vi "DWF Dig Tristate Lines.vi"(0 "Instrument Handle In":u32, 5 "Lines":string, 11 "Error In":errorcluster caption="Error In (no error)") -> (4 "Instrument Handle Out":u32, 15 "Error Out":errorcluster)   [LabVIEW 2015, in "DigilentWF.lvlib"]
doc: "Sets all specified lines to a high-impedance state."
uses:
  <vilib>/DigilentWF/DigilentWF.lvlib
  dwf.dll
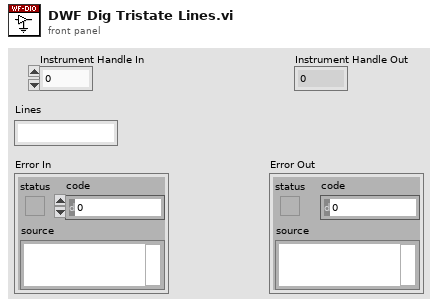
[diagram p1: front panel]
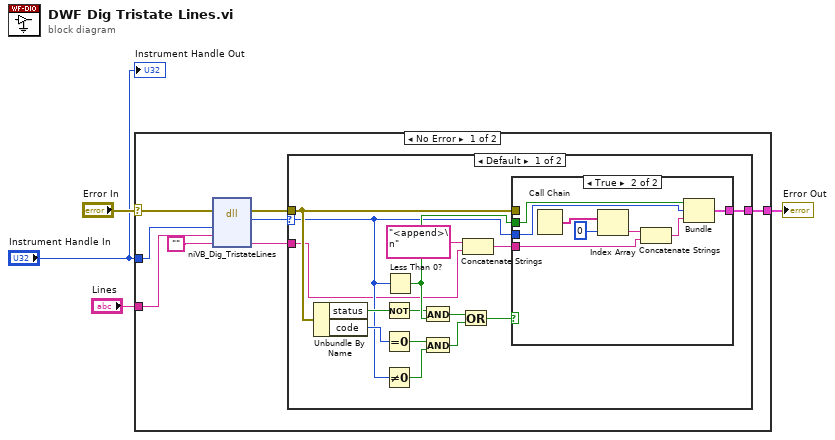
[diagram p0: block diagram]
diagram:
  n1 = case "outter_case" shown="No Error" "Error In" {
    selector: "Error In" -> [w9 w38]
    tunnel: [w12 w38] -> w3
    tunnel: "Instrument Handle In" -> [w8 _]
    tunnel: "Lines" -> [w7 _]
    frame No Error {
      n2 = dll-call lib="dwf.*" fn="niVB_Dig_TristateLines"(error in=w9, "instrumentHandle"=w8, "lines"=w7, "szError"="") -> (error out=w11:errorcluster, "return type"=w10:u32, "szError"=w5:string)  [unwired: 4 in, 1 out]
      n3 = case "inner_case" shown="Default" w10 {
        selector: w10 -> [w17 _]
        tunnel: w11 -> [w18 w37]
        tunnel: [w14 w37] -> w12
        tunnel: w5 -> [w13 _]
        frame Default {
          n4 = Unbundle By Name(w18) -> ("status"=w22:bool, "code"=w26:i32)
          n5 = Not(x=w22) -> (.not. x?=w25:bool)
          n6 = Equal To 0?(x=w26) -> (x = 0?=w21:bool)
          n7 = Not Equal To 0?(x=w17) -> (x != 0?=w24:bool)
          n8 = Less Than 0?(x=w17) -> (x < 0?=w27:bool)
          n9 = And(x=w25, y=w27) -> (x .and. y?=w23:bool)
          n10 = And(x=w21, y=w24) -> (x .and. y?=w20:bool)
          n11 = Or(x=w23, y=w20) -> (x .or. y?=w19:bool)
          n12 = Concatenate Strings("<append>\n" ("string"), w13) -> (w16:string)
          n13 = case shown="True" w19 {
            tunnel: [w28 w35] -> w14
            tunnel: w17 -> [_ w34]
            tunnel: w27 -> [_ w33]
            tunnel: w18 -> [w28 _]
            tunnel: w16 -> [_ w29]
            frame False {
            }
            frame True {
              n14 = Call Chain() -> (call chain=w32:string[])
              n15 = Index Array(array=w32, index=0) -> (element=w31:string)
              n16 = Concatenate Strings(w31, w29) -> (w36:string)
              n17 = Bundle(w33, "return type"=w34, w36) -> (w35:cluster{bool, "return type":u32, string})  [unwired: 1 out]
            }
          }
        }
        frame 0 {
        }
      }
    }
    frame Error {
    }
  }
  "Error Out" <- w3
  "Instrument Handle Out" <- "Instrument Handle In"
